vi "_Parse ACLR Limit Check Result.vi"(8 "error in (no error)":errorcluster, 10 "Input String":string, 11 "VISA resource name":refnum<visa-resource-name>) -> (0 "error out":errorcluster, 1 "Limit Check Results":T1, 2 "Reliability":i32, 3 "VISA resource name out":refnum<visa-resource-name>)   [LabVIEW 2015, in "Rohde&Schwarz CMXP NR FR2 Measurement.lvlib"]
uses:
  <instrlib>/Rohde&Schwarz CMXP NR FR2 Measurement/Rohde&Schwarz CMXP NR FR2 Measurement.lvlib
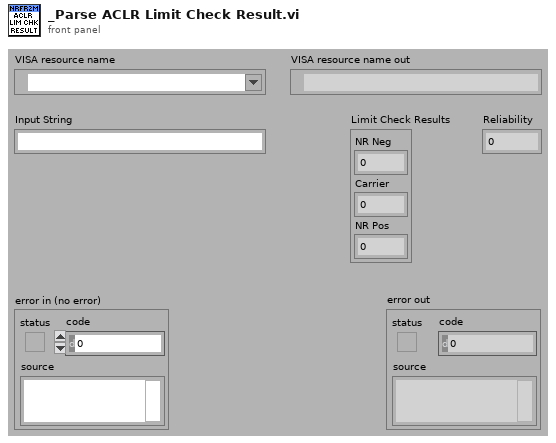
[diagram p1: front panel]
types:
  T1 = cluster{"NR Neg":i32, "Carrier":i32, "NR Pos":i32}
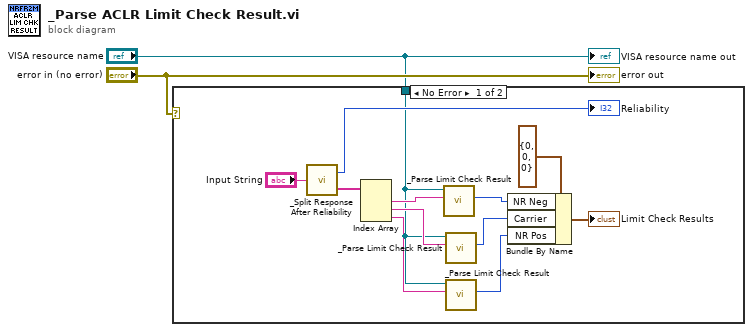
[diagram p0: block diagram]
diagram:
  n1 = case shown="No Error" "error in (no error)" {
    tunnel: "VISA resource name" -> [w3 _]
    frame No Error {
      n2 = call <instrlib>:"_Split Response After Reliability.vi"("Input String"="Input String") -> ("Response out"=w7:string[], "Reliability out"=→"Reliability":i32)
      n3 = Index Array(array=w7) -> (element #1=w6:string, element #2=w5:string, element #3=w4:string)  [unwired: 3 in]
      n4 = call <instrlib>:"_Parse Limit Check Result.vi"("String Value In"=w6, "VISA resource name"=w3) -> ("Limit Check Value"=w13:i32)  [unwired: 7 in, 2 out]
      n5 = call <instrlib>:"_Parse Limit Check Result.vi"("String Value In"=w5, "VISA resource name"=w3) -> ("Limit Check Value"=w12:i32)  [unwired: 7 in, 2 out]
      n6 = call <instrlib>:"_Parse Limit Check Result.vi"("String Value In"=w4, "VISA resource name"=w3) -> ("Limit Check Value"=w11:i32)  [unwired: 7 in, 2 out]
      n7 = Bundle By Name(cluster=T1 {"NR Neg"=0, "Carrier"=0, "NR Pos"=0} ("Limit Check Results"), "NR Neg"=w13, "Carrier"=w12, "NR Pos"=w11) -> (→"Limit Check Results":T1)
    }
    frame Error {
    }
  }
  "VISA resource name out" <- "VISA resource name"
  "error out" <- "error in (no error)"
